vi "Part 2 Replace Array Subset & Insert Into Array.vi"() -> ()   [LabVIEW 2020]
panel:
  in  "new element/subarray 2":dbl
  in  "new element/subarray":dbl
  out "output array 2":dbl[](array[numeric])
  out "output array":dbl[](array[numeric])
  in  "array":dbl[](array[numeric])
  # "Replace Array Subset & Insert Into Array"
  # "0          1         2"
  # "Replace Array Subset"
  # "0           1         2"
  # "Insert Into Array"
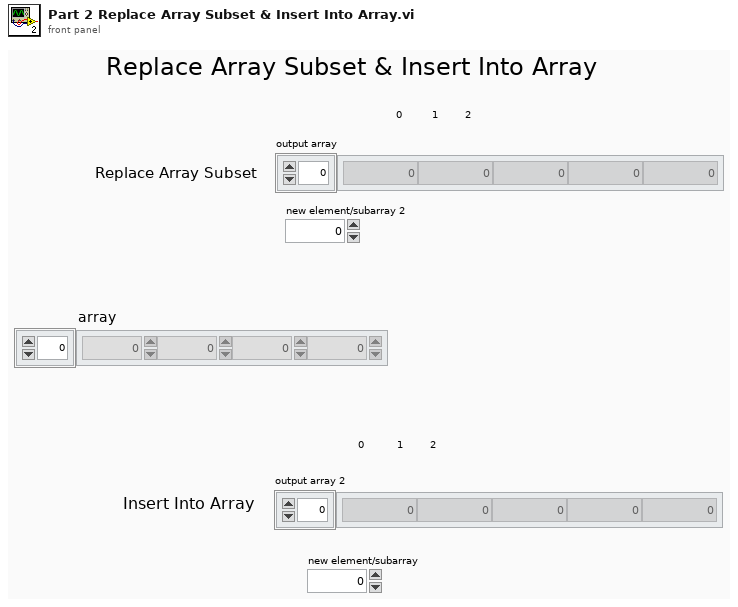
[diagram p1: front panel]
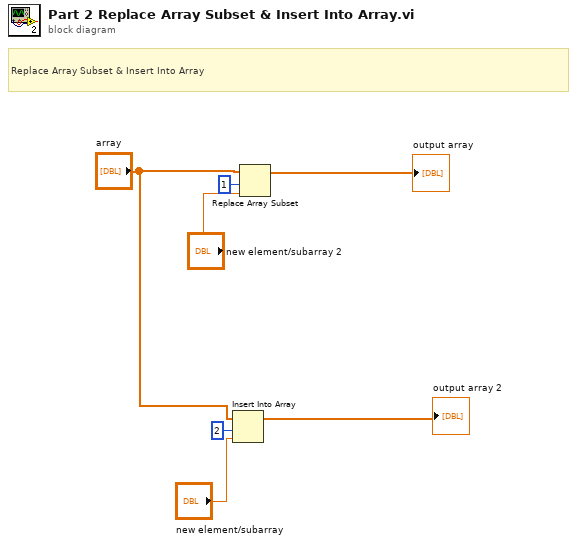
[diagram p0: block diagram]
diagram:
  # "Replace Array Subset & Insert Into Array"
  n1 = Insert Into Array "Insert Into Array"(array="array", index=2, new element="new element/subarray") -> (→"output array 2":dbl[])
  n2 = Replace Array Subset "Replace Array Subset"(array="array", new element="new element/subarray 2", index=1) -> (→"output array":dbl[])
